vi "Balance Movement Slow.vi"(6 "range":u16=45, 7 "Value":u16=1710, 8 "error out 2":errorcluster, 9 "Speed":dbl=50.0, 10 "Move":T1(ring), 11 "FPGA VI Reference Out":refnum<k20>) -> (0 "error out":errorcluster, 3 "FPGA VI Reference Out 2":refnum<k20>)   [LabVIEW 2019]
uses:
  <vilib>/Platform/TimedLoop/XDataNode/timing_clust.ctl
  <vilib>/Platform/TimedLoop/XDataNode/nitl_modes.ctl
  <vilib>/Platform/TimedLoop/XDataNode/wakeup.ctl
  <vilib>/robotics/Steering/Mecanum Wheel/Roller Orientation.ctl
  <vilib>/robotics/Steering/Wheel/Wheel Parameters.ctl
  <vilib>/robotics/Steering/Wheel/Rotation Direction.ctl
  <vilib>/robotics/Steering/Mecanum Steering Frame/NI_Robotics_Mecanum Steering Frame.lvclass
  C:/Program Files (x86)/National Instruments/LabVIEW 2019/vi.lib/robotics/Steering/Steering Frame/NI_Robotics_Steering Frame.lvclass
  <vilib>/robotics/Steering/Mecanum Wheel/Create Mecanum Wheel.vi
  <vilib>/robotics/Steering/Mecanum Steering Frame/Create Mecanum Steering Frame.vi
  <vilib>/robotics/Steering/Steering Frame/Apply Steering Frame Velocity to Motors.vi
  <vilib>/Utility/error.llb/Error Cluster From Error Code.vi
  <vilib>/rvi/errors/niLvFpgaAdjustHostInterfaceError.vi
  <vilib>/platform/TimedLoop/XDataNode/XDataNode.xnode
  <vilib>/robotics/Steering/Create Steering Frame/NI_Robotics_Create Steering Frame.xnode
  <vilib>/robotics/Steering/Class Type Definitions/Mecanum Steering Frame.ctl
  <vilib>/rvi/interface/nirviReadWriteControl/nirviReadWriteControl.xnode
  <vilib>/rvi/interface/Simulation/niFpgaSimulationCallBeginRW.vi
  <vilib>/Platform/TimedLoop/XDataNode/XDNodeRunTimeDep.lvlib
  <vilib>/robotics/Steering/Class Type Definitions/NI_Robotics_Steering Class Types.lvlib
  <vilib>/robotics/Steering/Mecanum Wheel/NI_Robotics_Mecanum Wheel.lvclass
  <vilib>/robotics/Steering/Wheel/NI_Robotics_Wheel.lvclass
  <vilib>/robotics/Steering/Steering Frame/NI_Robotics_Steering Frame.lvclass
  NiFpgaLv.dll
  C:/Program Files (x86)/National Instruments/LabVIEW 2019/vi.lib/robotics/Steering/Special Steering Frame/NI_Robotics_Special Steering Frame.lvclass
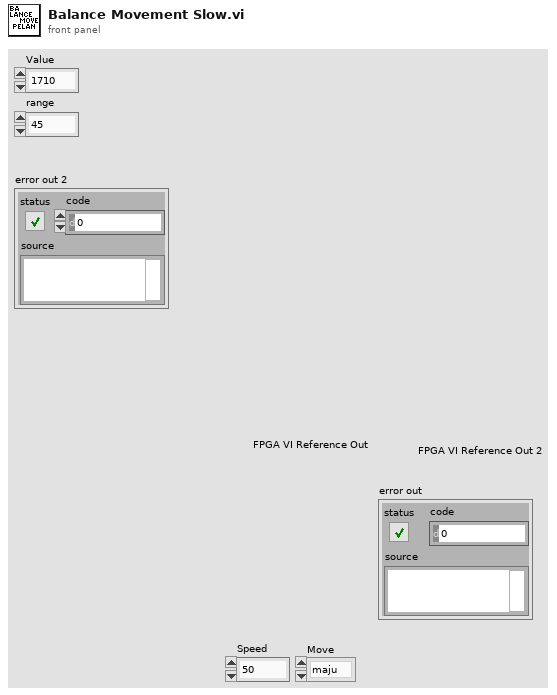
[diagram p1: front panel]
types:
  T1 = enum16{"maju", "mundur", "kanan", "kiri", "atas kanan", "atas kiri", "bawah kanan", "bawah kiri", "putar kanan", "putar kiri"}
  T2 = typedef "NI_Robotics_Steering Class Types.lvlib/Mecanum Steering Frame.ctl" = refnum<class "NI_Robotics_Mecanum Steering Frame.lvclass">
  T3 = typedef "XDNodeRunTimeDep.lvlib/timing_clust.ctl" = cluster{"Expected End [f-1]":u64, "Actual End [f-1]":u64, "Finished Late? [f-1]":bool, "Expected End [i-1]":u64, "Actual End [i-1]":u64, "Finished Late? [i-1]":bool, "Expected Start [i]":u64, "Actual Start [i]":u64, "Expected Start [f]":u64, "Actual Start [f]":u64, "Source Name":string, "Structure Name":string, "Period":i64, "Deadline":i64, "Offset":i64, "Start":i64, "Priority":i32, "Timeout":i32, "Mode":T4, "Wakeup Reason":T5, "Error":errorcluster, "Source Type":string, "Secondary Source Type":string, "Global End Time":u64, "Global Start Time":u64, "Frame Duration":u64, "Iteration Duration":u64, "Assigned CPU":i32, "I/O Scan Engine Mode":u32}
  T4 = typedef "XDNodeRunTimeDep.lvlib/nitl_modes.ctl" = enum32{"No Change", "Process missed periods, maintain original phase", "Discard missed periods, maintain original phase", "Process missed periods, ignore original phase", "Discard missed periods, ignore original phase"}
  T5 = typedef "XDNodeRunTimeDep.lvlib/wakeup.ctl" = enum32{"Normal", "Aborted", "Asynchronous wakeup", "Timing source error", "Timed loop error", "Timeout"}
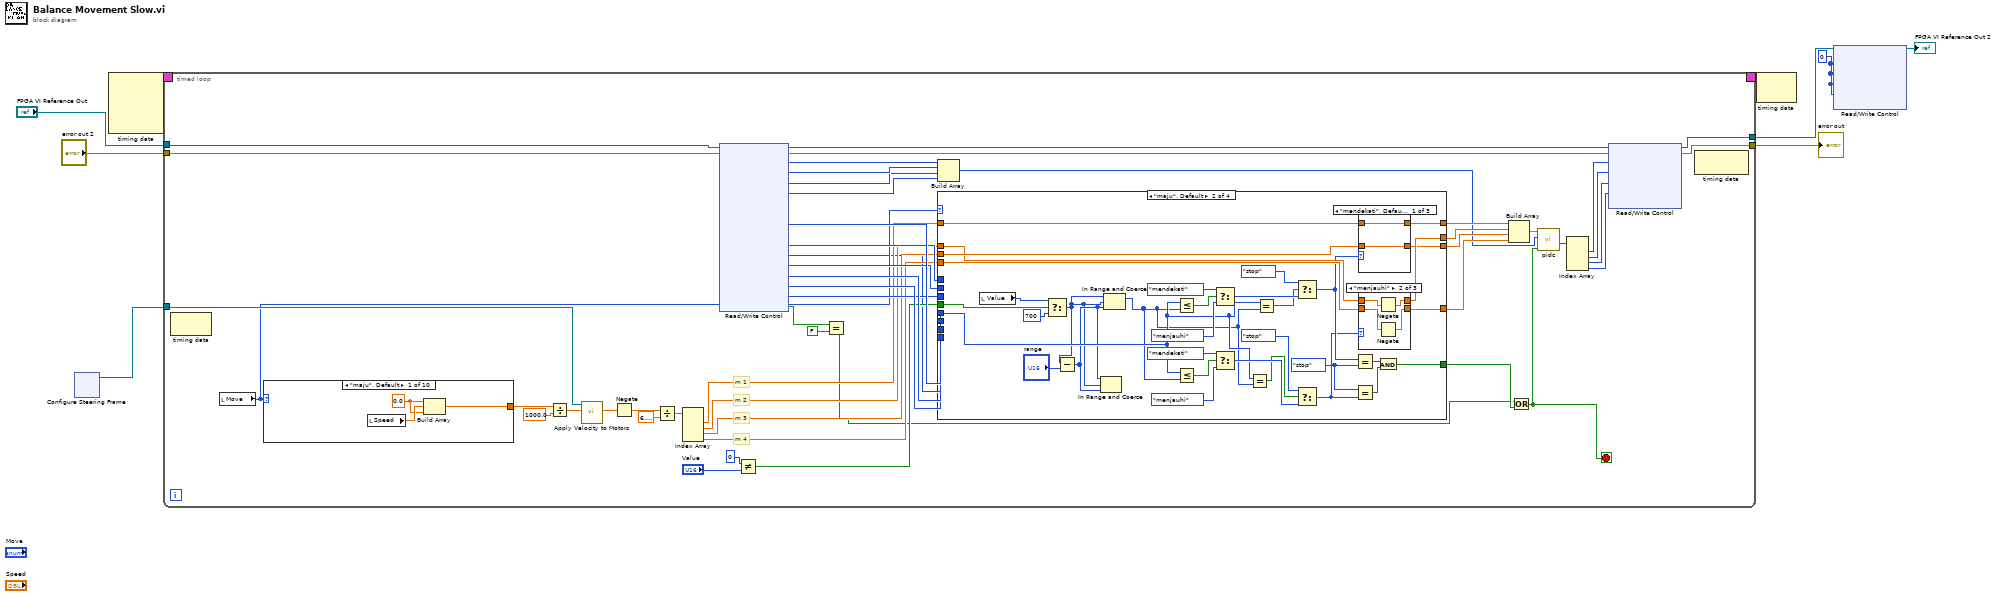
[diagram p0: block diagram]
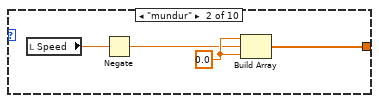
[diagram p2: hidden frame]
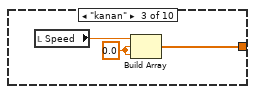
[diagram p3: hidden frame]
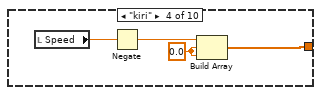
[diagram p4: hidden frame]
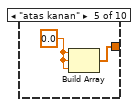
[diagram p5: hidden frame]
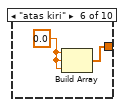
[diagram p6: hidden frame]
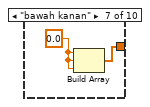
[diagram p7: hidden frame]
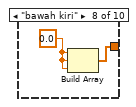
[diagram p8: hidden frame]
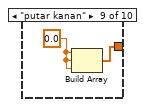
[diagram p9: hidden frame]
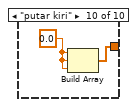
[diagram p10: hidden frame]
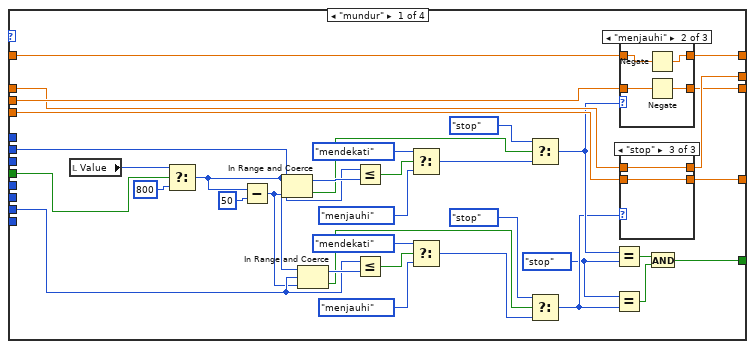
[diagram p11: hidden frame]
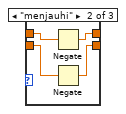
[diagram p13: hidden frame]
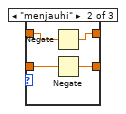
[diagram p18: hidden frame]
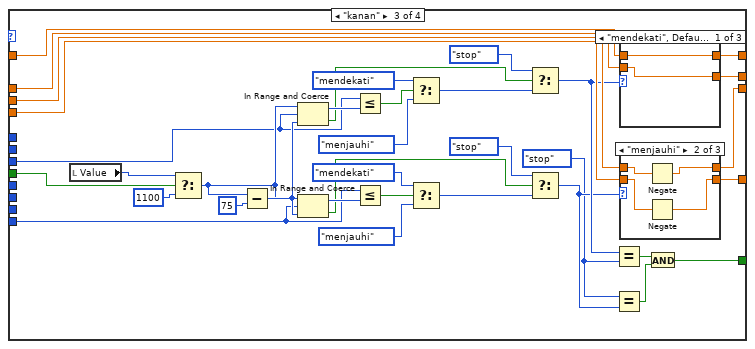
[diagram p20: hidden frame]
diagram:
  w2 = i16 0 ("M1")
  n1 = xnode ("Configure Steering Frame")() -> ("mecanum steering frame out"=w5:T2)  [unwired: 1 in, 1 out]
  n2 = node-c288() -> (w7:T3)  [unwired: 4 in]
  n3 = timed-loop {
    timing: w7 -> [_]
    timing-out: [_] -> w6
    tunnel: "FPGA VI Reference Out" -> [w58]
    tunnel: "error out 2" -> [w54]
    tunnel: [w57] -> w8
    tunnel: [w56] -> w9
    tunnel: w5 -> [w52]
    stop <- w13 stop-if-true
    # "m 4"
    # "m 3"
    # "m 2"
    # "m 1"
    n4 = node-c288() -> ()  [unwired: 1 in, 1 out]
    n5 = local read "Move"() -> (w24:T1)
    n6 = case shown="\"maju\", Default" w24 {
      tunnel: [w59 w63 w67 w71 w74 w76 w78 w80 w82 w84] -> w25
      frame "maju", Default {
        w60 = 0.0 ("element")
        n7 = local read "Speed"() -> (w61:dbl)
        n8 = Build Array(w60, w61, w60) -> (w59:dbl[])
      }
      frame "mundur" {
        w64 = 0.0 ("element")
        n9 = local read "Speed"() -> (w65:dbl)
        n10 = Negate(x=w65) -> (-x=w62:dbl)
        n11 = Build Array(w64, w62, w64) -> (w63:dbl[])
      }
      frame "kanan" {
        w66 = 0.0 ("element")
        n12 = local read "Speed"() -> (w68:dbl)
        n13 = Build Array(w68, w66, w66) -> (w67:dbl[])
      }
      frame "kiri" {
        w69 = 0.0 ("element")
        n14 = local read "Speed"() -> (w72:dbl)
        n15 = Negate(x=w72) -> (-x=w70:dbl)
        n16 = Build Array(w70, w69, w69) -> (w71:dbl[])
      }
      frame "atas kanan" {
        w73 = 0.0 ("element")
        n17 = Build Array(w73, w73, w73) -> (w74:dbl[])
      }
      frame "atas kiri" {
        w75 = 0.0 ("element")
        n18 = Build Array(w75, w75, w75) -> (w76:dbl[])
      }
      frame "bawah kanan" {
        w77 = 0.0 ("element")
        n19 = Build Array(w77, w77, w77) -> (w78:dbl[])
      }
      frame "bawah kiri" {
        w79 = 0.0 ("element")
        n20 = Build Array(w79, w79, w79) -> (w80:dbl[])
      }
      frame "putar kanan" {
        w81 = 0.0 ("element")
        n21 = Build Array(w81, w81, w81) -> (w82:dbl[])
      }
      frame "putar kiri" {
        w83 = 0.0 ("element")
        n22 = Build Array(w83, w83, w83) -> (w84:dbl[])
      }
    }
    n23 = Divide(x=w25, y=1000.0) -> (x/y=w20:dbl[])
    n24 = call-poly <vilib>:"Apply Velocity to Motors.vi"("steering frame velocity"=w20, "steering frame in"=w52) -> ("ccw motor velocity setpoints"=w50:dbl[])  [unwired: 5 in, 4 out]
    n25 = Negate(x=w50) -> (-x=w51:dbl[])
    n26 = Divide(x=w51, y=6.283185307179586) -> (x/y=w41:dbl[])
    n27 = Index Array(array=w41) -> (element #1=w33:dbl, element #2=w32:dbl, element #3=w31:dbl, element #4=w30:dbl)  [unwired: 4 in]
    n28 = xnode "Read/Write Control"("FPGA VI Reference In"=w58, "error in"=w54) -> ("FPGA VI Reference Out"=w55:refnum<k20>, "error out"=w53:errorcluster, "ENC M1"=w49:i32, "ENC M2"=w48:i32, "ENC M3"=w47:i32, "ENC M4"=w46:i32, "IR 1"=w39:u16, "IR 3"=w38:u16, "IR 4"=w15:u16, "IR 5"=w37:u16, "IR 6"=w36:u16, "IR 7"=w35:u16, "IR 8"=w34:u16, "START BUTTON"=w12:bool)  [unwired: 3 out]
    n29 = Not Equal?(x=u16 0, y="Value") -> (x != y?=w16:bool)
    n30 = Equal?(x=w12, y=FALSE) -> (x = y?=w10:bool)
    n31 = Build Array(w49, w48, w47, w46) -> (w22:i32[])
    n32 = case shown="\"maju\", Default" w24 {
      tunnel: w39 -> [_ w143 _ _]
      tunnel: w38 -> [_ _ _ w238]
      tunnel: w15 -> [_ _ _ w237]
      tunnel: w37 -> [w119 _ _ _]
      tunnel: w36 -> [w107 _ _ _]
      tunnel: w35 -> [_ _ w187 _]
      tunnel: w34 -> [_ _ w188 _]
      tunnel: w33 -> [w106 w160 w208 w260]
      tunnel: w32 -> [w104 w158 w207 w259]
      tunnel: w31 -> [w105 w159 w206 w258]
      tunnel: w30 -> [w103 w157 w205 w257]
      tunnel: [w99 w153 w204 w256] -> w29
      tunnel: [w101 w155 w203 w255] -> w28
      tunnel: [w100 w154 w202 w254] -> w27
      tunnel: [w102 w156 w201 w253] -> w26
      tunnel: [w92 w147 w198 w247] -> w14
      tunnel: w16 -> [w85 w144 w189 w239]
      frame "mundur" {
        w91 = enum16{"mendekati", "menjauhi", "stop", "start"}."stop" ("t")
        n33 = local read "Value"() -> (w90:u16)
        n34 = Select(t=w90, s=w85, f=u16 800) -> (s? t:f=w86:u16)
        n35 = Subtract(x=w86, y=u16 50 ("upper limit")) -> (x-y=w87:u16)
        n36 = In Range and Coerce(upper limit=w86, x=w119, lower limit=w87) -> (coerced(x)=w120:u16, In Range?=w114:bool)
        n37 = In Range and Coerce(upper limit=w86, x=w107, lower limit=w87) -> (coerced(x)=w113:u16, In Range?=w108:bool)
        n38 = Less Or Equal?(x=w119, y=w120) -> (x <= y?=w115:bool)
        n39 = Less Or Equal?(x=w107, y=w113) -> (x <= y?=w109:bool)
        n40 = Select(t=enum16{"mendekati", "menjauhi", "stop", "start"}."mendekati", s=w115, f=enum16{"mendekati", "menjauhi", "stop", "start"}."menjauhi") -> (s? t:f=w117:enum16{"mendekati", "menjauhi", "stop", "start"})
        n41 = Select(t=enum16{"mendekati", "menjauhi", "stop", "start"}."mendekati", s=w109, f=enum16{"mendekati", "menjauhi", "stop", "start"}."menjauhi") -> (s? t:f=w111:enum16{"mendekati", "menjauhi", "stop", "start"})
        n42 = Select(t=enum16{"mendekati", "menjauhi", "stop", "start"}."stop", s=w114, f=w117) -> (s? t:f=w94:enum16{"mendekati", "menjauhi", "stop", "start"})
        n43 = Select(t=enum16{"mendekati", "menjauhi", "stop", "start"}."stop", s=w108, f=w111) -> (s? t:f=w93:enum16{"mendekati", "menjauhi", "stop", "start"})
        n44 = Equal?(x=w94, y=w91) -> (x = y?=w98:bool)
        n45 = Equal?(x=w91, y=w93) -> (x = y?=w97:bool)
        n46 = case shown="\"menjauhi\"" w94 {
          tunnel: w106 -> [w130 w134 w136]
          tunnel: w105 -> [w129 w132 w135]
          tunnel: [w130 w133 w136] -> w99
          tunnel: [w129 w131 w135] -> w100
          frame "mendekati", Default {
          }
          frame "menjauhi" {
            n47 = Negate(x=w134) -> (-x=w133:dbl)
            n48 = Negate(x=w132) -> (-x=w131:dbl)
          }
          frame "stop" {
          }
        }
        n49 = case shown="\"stop\"" w93 {
          tunnel: w104 -> [w122 w126 w128]
          tunnel: w103 -> [w121 w125 w127]
          tunnel: [w121 w124 w127] -> w102
          tunnel: [w122 w123 w128] -> w101
          frame "mendekati", Default {
          }
          frame "menjauhi" {
            n50 = Negate(x=w126) -> (-x=w123:dbl)
            n51 = Negate(x=w125) -> (-x=w124:dbl)
          }
          frame "stop" {
          }
        }
        n52 = And(x=w98, y=w97) -> (x .and. y?=w92:bool)
      }
      frame "maju", Default {
        w148 = enum16{"mendekati", "menjauhi", "stop", "start"}."stop" ("t")
        n53 = local read "Value"() -> (w146:u16)
        n54 = Select(t=w146, s=w144, f=u16 700) -> (s? t:f=w139:u16)
        n55 = Subtract(x=w139, y="range") -> (x-y=w140:u16)
        n56 = In Range and Coerce(upper limit=w140, x=w139, lower limit=w140) -> ()  [unwired: 2 out]
        n57 = In Range and Coerce(upper limit=w139, x=w139, lower limit=w140) -> (coerced(x)=w138:u16)  [unwired: 1 out]
        n58 = Less Or Equal?(x=w143, y=w138) -> (x <= y?=w166:bool)
        n59 = Less Or Equal?(x=w143, y=w138) -> (x <= y?=w161:bool)
        n60 = Select(t=enum16{"mendekati", "menjauhi", "stop", "start"}."mendekati", s=w166, f=enum16{"mendekati", "menjauhi", "stop", "start"}."menjauhi") -> (s? t:f=w169:enum16{"mendekati", "menjauhi", "stop", "start"})
        n61 = Select(t=enum16{"mendekati", "menjauhi", "stop", "start"}."mendekati", s=w161, f=enum16{"mendekati", "menjauhi", "stop", "start"}."menjauhi") -> (s? t:f=w164:enum16{"mendekati", "menjauhi", "stop", "start"})
        n62 = Equal?(x=w143, y=w138) -> (x = y?=w142:bool)
        n63 = Equal?(x=w143, y=w138) -> (x = y?=w141:bool)
        n64 = Select(t=enum16{"mendekati", "menjauhi", "stop", "start"}."stop", s=w141, f=w169) -> (s? t:f=w150:enum16{"mendekati", "menjauhi", "stop", "start"})
        n65 = Select(t=enum16{"mendekati", "menjauhi", "stop", "start"}."stop", s=w142, f=w164) -> (s? t:f=w149:enum16{"mendekati", "menjauhi", "stop", "start"})
        n66 = Equal?(x=w150, y=w148) -> (x = y?=w152:bool)
        n67 = Equal?(x=w148, y=w149) -> (x = y?=w151:bool)
        n68 = case shown="\"mendekati\", Default" w150 {
          tunnel: w160 -> [w180 w184 w186]
          tunnel: w159 -> [w179 w182 w185]
          tunnel: [w180 w183 w186] -> w153
          tunnel: [w179 w181 w185] -> w154
          frame "mendekati", Default {
          }
          frame "menjauhi" {
            n69 = Negate(x=w184) -> (-x=w183:dbl)
            n70 = Negate(x=w182) -> (-x=w181:dbl)
          }
          frame "stop" {
          }
        }
        n71 = case shown="\"menjauhi\"" w149 {
          tunnel: w158 -> [w172 w176 w178]
          tunnel: w157 -> [w171 w175 w177]
          tunnel: [w171 w174 w177] -> w156
          tunnel: [w172 w173 w178] -> w155
          frame "mendekati", Default {
          }
          frame "menjauhi" {
            n72 = Negate(x=w176) -> (-x=w173:dbl)
            n73 = Negate(x=w175) -> (-x=w174:dbl)
          }
          frame "stop" {
          }
        }
        n74 = And(x=w152, y=w151) -> (x .and. y?=w147:bool)
      }
      frame "kanan" {
        w195 = enum16{"mendekati", "menjauhi", "stop", "start"}."stop" ("t")
        n75 = local read "Value"() -> (w194:u16)
        n76 = Select(t=w194, s=w189, f=u16 1100) -> (s? t:f=w190:u16)
        n77 = Subtract(x=w190, y=u16 75) -> (x-y=w191:u16)
        n78 = In Range and Coerce(upper limit=w190, x=w188, lower limit=w191) -> (coerced(x)=w222:u16, In Range?=w216:bool)
        n79 = In Range and Coerce(upper limit=w190, x=w187, lower limit=w191) -> (coerced(x)=w215:u16, In Range?=w209:bool)
        n80 = Less Or Equal?(x=w188, y=w222) -> (x <= y?=w217:bool)
        n81 = Less Or Equal?(x=w187, y=w215) -> (x <= y?=w210:bool)
        n82 = Select(t=enum16{"mendekati", "menjauhi", "stop", "start"}."mendekati", s=w217, f=enum16{"mendekati", "menjauhi", "stop", "start"}."menjauhi") -> (s? t:f=w220:enum16{"mendekati", "menjauhi", "stop", "start"})
        n83 = Select(t=enum16{"mendekati", "menjauhi", "stop", "start"}."mendekati", s=w210, f=enum16{"mendekati", "menjauhi", "stop", "start"}."menjauhi") -> (s? t:f=w213:enum16{"mendekati", "menjauhi", "stop", "start"})
        n84 = Select(t=enum16{"mendekati", "menjauhi", "stop", "start"}."stop", s=w216, f=w220) -> (s? t:f=w197:enum16{"mendekati", "menjauhi", "stop", "start"})
        n85 = Select(t=enum16{"mendekati", "menjauhi", "stop", "start"}."stop", s=w209, f=w213) -> (s? t:f=w196:enum16{"mendekati", "menjauhi", "stop", "start"})
        n86 = Equal?(x=w197, y=w195) -> (x = y?=w200:bool)
        n87 = Equal?(x=w195, y=w196) -> (x = y?=w199:bool)
        n88 = case shown="\"mendekati\", Default" w197 {
          tunnel: w208 -> [w231 w235 _]
          tunnel: w207 -> [w230 w233 _]
          tunnel: [w231 w234 w236] -> w204
          tunnel: [w230 w232 w236] -> w203
          frame "mendekati", Default {
          }
          frame "menjauhi" {
            n89 = Negate(x=w235) -> (-x=w234:dbl)
            n90 = Negate(x=w233) -> (-x=w232:dbl)
          }
          frame "stop" {
            w236 = 0.0
          }
        }
        n91 = case shown="\"menjauhi\"" w196 {
          tunnel: w206 -> [w224 w228 _]
          tunnel: w205 -> [w223 w227 _]
          tunnel: [w223 w226 w229] -> w201
          tunnel: [w224 w225 w229] -> w202
          frame "mendekati", Default {
          }
          frame "menjauhi" {
            n92 = Negate(x=w228) -> (-x=w225:dbl)
            n93 = Negate(x=w227) -> (-x=w226:dbl)
          }
          frame "stop" {
            w229 = 0.0
          }
        }
        n94 = And(x=w200, y=w199) -> (x .and. y?=w198:bool)
      }
      frame "kiri" {
        w250 = enum16{"mendekati", "menjauhi", "stop", "start"}."stop" ("t")
        n95 = local read "Value"() -> (w244:u16)
        n96 = Select(t=w244, s=w239, f=u16 1100) -> (s? t:f=w240:u16)
        n97 = Subtract(x=w240, y=u16 75) -> (x-y=w241:u16)
        n98 = In Range and Coerce(upper limit=w240, x=w238, lower limit=w241) -> (coerced(x)=w272:u16, In Range?=w267:bool)
        n99 = In Range and Coerce(upper limit=w240, x=w237, lower limit=w241) -> (coerced(x)=w266:u16, In Range?=w261:bool)
        n100 = Less Or Equal?(x=w238, y=w272) -> (x <= y?=w268:bool)
        n101 = Less Or Equal?(x=w237, y=w266) -> (x <= y?=w262:bool)
        n102 = Select(t=enum16{"mendekati", "menjauhi", "stop", "start"}."mendekati", s=w268, f=enum16{"mendekati", "menjauhi", "stop", "start"}."menjauhi") -> (s? t:f=w270:enum16{"mendekati", "menjauhi", "stop", "start"})
        n103 = Select(t=enum16{"mendekati", "menjauhi", "stop", "start"}."mendekati", s=w262, f=enum16{"mendekati", "menjauhi", "stop", "start"}."menjauhi") -> (s? t:f=w264:enum16{"mendekati", "menjauhi", "stop", "start"})
        n104 = Select(t=enum16{"mendekati", "menjauhi", "stop", "start"}."stop", s=w267, f=w270) -> (s? t:f=w246:enum16{"mendekati", "menjauhi", "stop", "start"})
        n105 = Select(t=enum16{"mendekati", "menjauhi", "stop", "start"}."stop", s=w261, f=w264) -> (s? t:f=w245:enum16{"mendekati", "menjauhi", "stop", "start"})
        n106 = Equal?(x=w246, y=w250) -> (x = y?=w249:bool)
        n107 = Equal?(x=w245, y=w250) -> (x = y?=w248:bool)
        n108 = case shown="\"menjauhi\"" w246 {
          tunnel: w260 -> [w281 w285 _]
          tunnel: w259 -> [w280 w283 _]
          tunnel: [w281 w284 w286] -> w256
          tunnel: [w280 w282 w286] -> w255
          frame "mendekati", Default {
          }
          frame "menjauhi" {
            n109 = Negate(x=w285) -> (-x=w284:dbl)
            n110 = Negate(x=w283) -> (-x=w282:dbl)
          }
          frame "stop" {
            w286 = 0.0
          }
        }
        n111 = case shown="\"menjauhi\"" w245 {
          tunnel: w258 -> [w274 w278 _]
          tunnel: w257 -> [w273 w277 _]
          tunnel: [w273 w276 w279] -> w253
          tunnel: [w274 w275 w279] -> w254
          frame "mendekati", Default {
          }
          frame "menjauhi" {
            n112 = Negate(x=w278) -> (-x=w275:dbl)
            n113 = Negate(x=w277) -> (-x=w276:dbl)
          }
          frame "stop" {
            w279 = 0.0
          }
        }
        n114 = And(x=w249, y=w248) -> (x .and. y?=w247:bool)
      }
    }
    n115 = Build Array(w29, w28, w27, w26) -> (w23:dbl[])
    n116 = Or(x=w10, y=w14) -> (x .or. y?=w13:bool)
    n117 = call "pidc.vi"("Stop"=w13, "input encoder 2"=w22, "input rps"=w23) -> ("Output duty cycle"=w21:i16[])  [unwired: 8 in]
    n118 = Index Array(array=w21) -> (element #1=w45:i16, element #2=w44:i16, element #3=w43:i16, element #4=w42:i16)  [unwired: 4 in]
    n119 = xnode "Read/Write Control"("FPGA VI Reference In"=w55, "error in"=w53, "M1"=w45, "M2"=w44, "M3"=w43, "M4"=w42) -> ("FPGA VI Reference Out"=w57:refnum<k20>, "error out"=w56:errorcluster)  [unwired: 1 in]
    n120 = node-c288() -> ()  [unwired: 1 in, 1 out]
  }
  "error out" <- w9
  n121 = node-c288(w6) -> ()  [unwired: 1 out]
  n122 = xnode "Read/Write Control"("FPGA VI Reference In"=w8, "M1"=w2, "M2"=w2, "M3"=w2, "M4"=w2) -> ("FPGA VI Reference Out"=→"FPGA VI Reference Out 2":refnum<k20>)  [unwired: 2 in, 1 out]
